vi "Initialization VI.vi"(8 "error in (no error)":errorcluster, 10 "Custom XML":string, 11 "Device Item Ref in":T1 format="%.0x") -> (0 "error out":errorcluster, 3 "Device Item Ref out":T1 format="%.0x")   [LabVIEW 2019, in "MD4Logger System Explorer.lvlib"]
uses:
  MD4Logger System Explorer.lvlib
  <vilib>/NI VeriStand/Custom Device API/Custom Device Item Ref.ctl
  <vilib>/NI VeriStand/Custom Device API/Custom Device Channel.ctl
  <vilib>/NI VeriStand/Custom Device API/Custom Device Channel Type.ctl
  Shared/Constants.vi
  <vilib>/NI/NI VeriStand Custom Device Import and Export Tool/ImportExport.lvlib
  Shared/MD4Logger Shared.lvlib
  <vilib>/NI VeriStand/Custom Device API/Custom Device API.lvlib
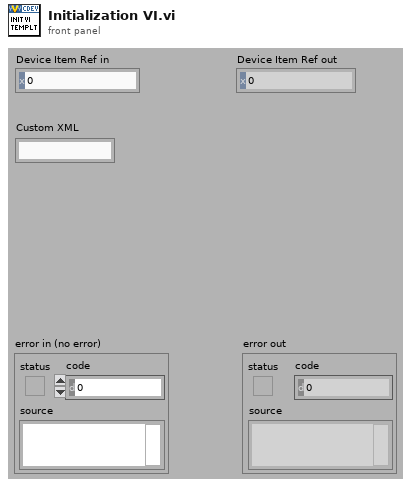
[diagram p1: front panel]
types:
  T1 = typedef "Custom Device API.lvlib/Custom Device Item Ref.ctl" = u64
  T2 = typedef "Custom Device API.lvlib/Custom Device Channel.ctl" = cluster{"Type":T3, "Units":string, "Default Value":dbl, "Faultable":bool, "Scalable":bool}
  T3 = typedef "Custom Device API.lvlib/Custom Device Channel Type.ctl" = enum16{"Input", "Output"}
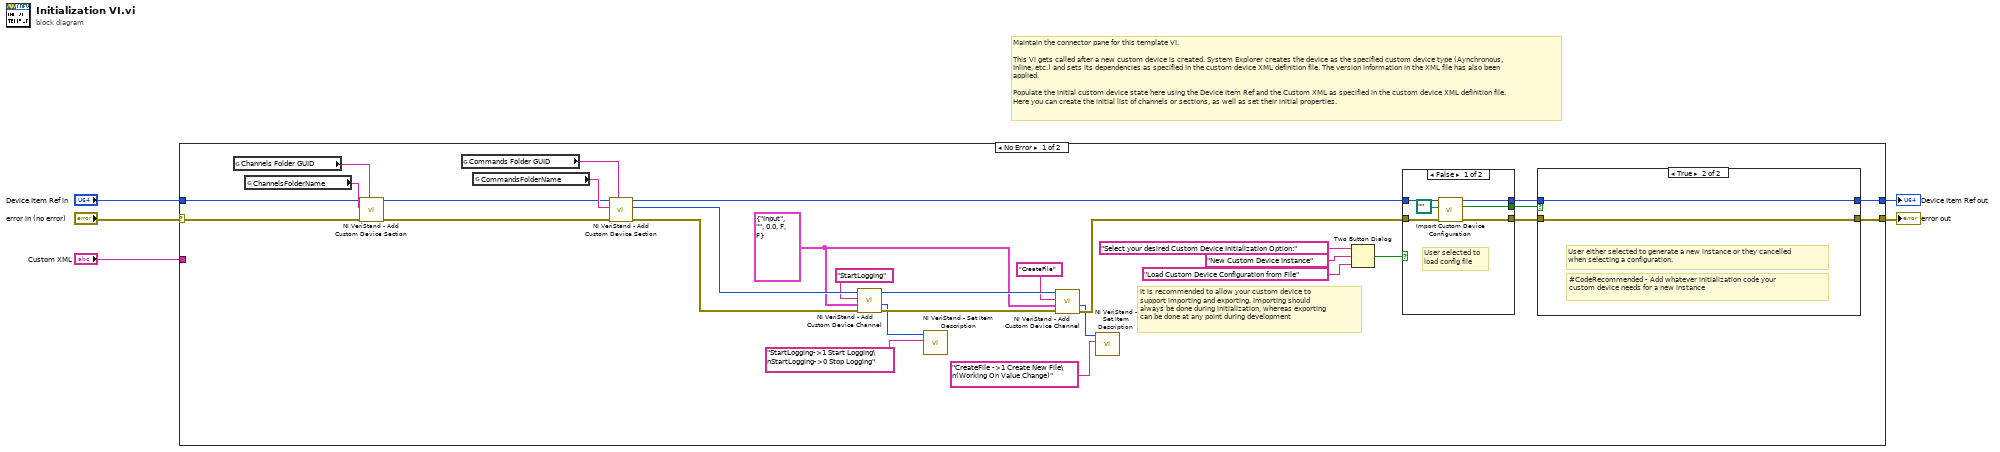
[diagram p0: block diagram]
diagram:
  # "Maintain the connector pane for this template VI.\n\nThis VI gets called after a new custom device is created. System Explorer creates the device as the specified custom device type (Aynchronous, Inline, etc.) and sets its dependencies as specified in the custom device XML definition file. The version information in the XML file has also been applied.\n\nPopulate the initial custom device state here using the Device Item Ref and the Custom XML as specified in the custom device XML definition file. Here you can create the initial list of channels or sections, as well as set their initial properties."
  n1 = case shown="No Error" "error in (no error)" {
    selector: "error in (no error)" -> [w15 w50]
    tunnel: [w28 w50] -> w5
    tunnel: [w27 w49] -> w3
    tunnel: "Device Item Ref in" -> [w16 w49]
    tunnel: "Custom XML" -> [_ _]
    frame No Error {
      w10 = T2 {"Type"=enum."Input", "Units"="", "Default Value"=0.0, "Faultable"=FALSE, "Scalable"=FALSE} ("Channel")
      # "It is recommended to allow your custom device to\nsupport importing and exporting. Importing should\nalways be done during initialization, whereas exporting\ncan be done at any point during development"
      n2 = global read "Constants.vi" "Channels Folder GUID"() -> (w26:string)
      n3 = global read "Constants.vi" "ChannelsFolderName"() -> (w25:string)
      n4 = call <vilib>:"NI VeriStand - Add Custom Device Section.vi"("GUID (Default Section)"=w26, "error in (no error)"=w15, "Section Name"=w25, "Parent Ref in"=w16) -> ("error out"=w13:errorcluster, "Parent Ref out"=w14:T1)  [unwired: 4 in, 2 out]
      n5 = global read "Constants.vi" "Commands Folder GUID"() -> (w24:string)
      n6 = global read "Constants.vi" "CommandsFolderName"() -> (w23:string)
      n7 = call <vilib>:"NI VeriStand - Add Custom Device Section.vi"("GUID (Default Section)"=w24, "error in (no error)"=w13, "Section Name"=w23, "Parent Ref in"=w14) -> ("error out"=w18:errorcluster, "Section Ptr"=w22:T1, "Parent Ref out"=w12:T1)  [unwired: 4 in, 1 out]
      n8 = call <vilib>:"NI VeriStand - Add Custom Device Channel.vi"("error in (no error)"=w18, "Channel"=w10, "Channel Name"="StartLogging", "Parent Ref in"=w22) -> ("error out"=w20:errorcluster, "Channel Ref"=w9:T1, "Parent Ref out"=w19:T1)  [unwired: 4 in, 1 out]
      n9 = call <vilib>:"NI VeriStand - Set Item Description.vi"("Description"="StartLogging->1 Start Logging\nStartLogging->0 Stop Logging", "Item Ref in"=w9) -> ()  [unwired: 7 in, 3 out]
      n10 = call <vilib>:"NI VeriStand - Add Custom Device Channel.vi"("error in (no error)"=w20, "Channel"=w10, "Channel Name"="CreateFile", "Parent Ref in"=w19) -> ("error out"=w11:errorcluster, "Channel Ref"=w7:T1)  [unwired: 4 in, 2 out]
      n11 = call <vilib>:"NI VeriStand - Set Item Description.vi"("Description"="CreateFile ->1 Create New File\n(Working On Value Change)", "Item Ref in"=w7) -> ()  [unwired: 7 in, 3 out]
      n12 = Two Button Dialog(message="Select your desired Custom Device Initialization Option:", 1:"Load Custom Device Configuration from File" ("F button name (\"Cancel\")"), 2:"New Custom Device Instance" ("T button name (\"OK\")")) -> (T button?=w32:bool)
      n13 = case shown="False" w32 {
        selector: w32 -> [_ w46]
        tunnel: w12 -> [w45 w48]
        tunnel: [w44 w48] -> w31
        tunnel: w11 -> [w42 w47]
        tunnel: [w41 w47] -> w29
        tunnel: [w40 w46] -> w30
        frame False {
          # "User selected to\nload config file"
          n14 = call <vilib>:"Import Custom Device Configuration.vi"("error in (no error)"=w42, "Path"=path "", "NodeID"=w45) -> ("error out"=w41:errorcluster, "cancelled"=w40:bool, "NodeID out"=w44:u64)  [unwired: 6 in]
        }
        frame True {
          # "User selected new\ncustom device. Do\nnothing in this case\nand handle new\ngeneration in the\nnext case structure"
        }
      }
      n15 = case shown="True" w30 {
        tunnel: w31 -> [w37 w38]
        tunnel: w29 -> [w36 w39]
        tunnel: [w36 w39] -> w28
        tunnel: [w37 w38] -> w27
        frame False {
          # "User selected to import from configuration and didn't cancel import"
        }
        frame True {
          # "#CodeRecommended - Add whatever initialization code your\ncustom device needs for a new instance"
          # "User either selected to generate a new instance or they cancelled\nwhen selecting a configuration."
        }
      }
    }
    frame Error {
    }
  }
  "error out" <- w5
  "Device Item Ref out" <- w3
